vi "Time Bar.vi"(10 "y":dbl=1.0) -> ()   [LabVIEW 2014]
panel:
  out "Slide":i64(slide) scale=0.0..2000.0
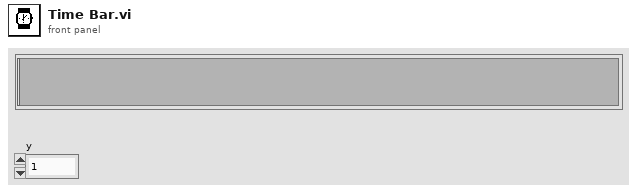
[diagram p1: front panel]
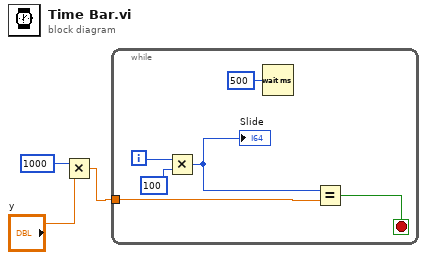
[diagram p0: block diagram]
diagram:
  n1 = Multiply(x=1000, y="y") -> (x*y=w1:dbl)
  n2 = while {
    tunnel: w1 -> [w4]
    i -> [w9]
    stop <- w6 stop-if-true
    n3 = Multiply(x=w9, y=100) -> (x*y=w5:i32)
    "Slide" <- w5
    n4 = Wait (ms)(milliseconds to wait=u32 500) -> ()  [unwired: 1 out]
    n5 = Equal?(x=w5, y=w4) -> (x = y?=w6:bool)
  }
